vi "JSON Delta Accel Update.vi"(9 "Delta JSON":string, 11 "input":T1={"type"="AI", "device"="", "name"="", "data"={"<init"=FALSE, "<range"=0.0, ">x"=0.0, ">y"=0.0, ">z"=0.0}}) -> (0 "error out":errorcluster, 3 "output":T1={"type"="AI", "device"="", "name"="", "data"={"<init"=FALSE, "<range"=0.0, ">x"=0.0, ">y"=0.0, ">z"=0.0}})   [LabVIEW 2019]
uses:
  Accel proto.ctl
  Accel Data proto.ctl
panel:
  out "JSON of original":string
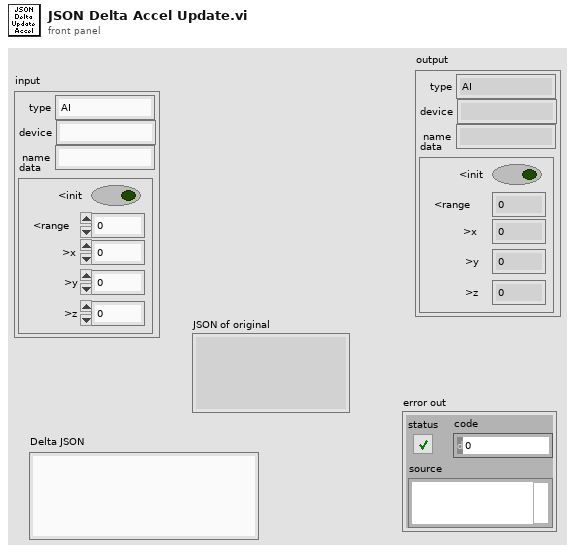
[diagram p1: front panel]
types:
  T1 = typedef "Accel proto.ctl" = cluster{"type":string, "device":string, "name":string, "data":T2}
  T2 = typedef "Accel Data proto.ctl" = cluster{"<init":bool, "<range":dbl, ">x":dbl, ">y":dbl, ">z":dbl}
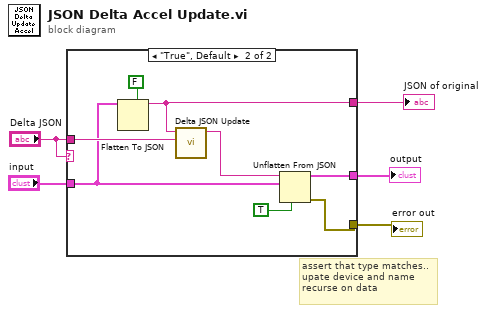
[diagram p0: block diagram]
diagram:
  # "assert that type matches..\nupate device and name\nrecurse on data"
  n1 = case shown="\"True\", Default" "Delta JSON" {
    tunnel: [_ w13] -> w5
    tunnel: "Delta JSON" -> [_ w11]
    tunnel: [_ w10] -> w4
    tunnel: "input" -> [w6 w8]
    tunnel: [w6 w7] -> w2
    frame "" {
    }
    frame "True", Default {
      n2 = Flatten To JSON(enable LabVIEW extensions? (T)=FALSE, anything=w8) -> (JSON string=w13:string)  [unwired: 1 in, 1 out]
      n3 = call "Delta JSON Update.vi"("Delta JSON"=w11, "JSON string in"=w13) -> ("JSON string out"=w12:string)  [unwired: 9 in]
      n4 = Unflatten From JSON(JSON string=w12, type and defaults=w8, default null elements? (F)=TRUE) -> (value=w7:T1, error out=w10:errorcluster)  [unwired: 4 in]
    }
  }
  "JSON of original" <- w5
  "error out" <- w4
  "output" <- w2
